vi "Initialize Attributes (public).vi"(8 "error in (no error)":errorcluster, 10 "Attribute Data":variant, 11 "CS++BaseActor in":refnum<class "CS++BaseActor.lvclass">) -> (0 "error out":errorcluster, 2 "Found?":bool, 3 "CS++BaseActor out":refnum<class "CS++BaseActor.lvclass">)   [LabVIEW 2013, in "CS++BaseActor.lvlib" / "CS++BaseActor.lvclass"]
doc: "Initialize object attribute.\n\nUnique resources should be allocated elsewhere!"
uses:
  CS++BaseActor.lvclass
  CS++BaseActor.lvclass/CS++BaseActor.ctl
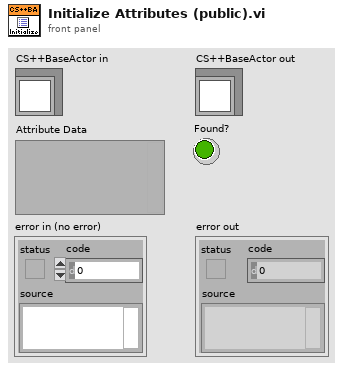
[diagram p1: front panel]
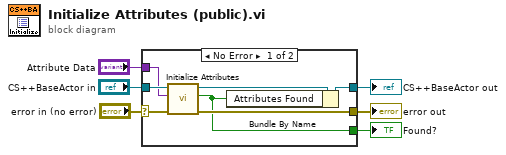
[diagram p0: block diagram]
diagram:
  n1 = case shown="No Error" "error in (no error)" {
    selector: "error in (no error)" -> [w13 w15]
    tunnel: [w12 w15] -> w5
    tunnel: [w8 w14] -> w3
    tunnel: "CS++BaseActor in" -> [w11 w14]
    tunnel: "Attribute Data" -> [w10 _]
    tunnel: [w7 _] -> w1
    frame No Error {
      n2 = call-dynamic "Initialize Attributes.vi"("error in (no error)"=w13, "Attribute Data"=w10, "CS++BaseActor in"=w11) -> ("error out"=w12:errorcluster, "Found?"=w7:bool, "CS++BaseActor out"=w9:refnum<class "CS++BaseActor.lvclass">)  [unwired: 6 in]
      n3 = Bundle By Name(cluster=w9, "Attributes Found"=w7) -> (w8:refnum<class "CS++BaseActor.lvclass">)
    }
    frame Error {
    }
  }
  "error out" <- w5
  "CS++BaseActor out" <- w3
  "Found?" <- w1
